vi "Initialization_ITC503_ver1.0.vi"(2 "error in":errorcluster, 3 "Temperature Control (ITC 503):":T1={"GPIB ADR"=0, "Change Heater?"={"Change Heater?"=FALSE, "Heater"=0}, "Change Temp?"={"Change Temp?"=FALSE, "Set Temp (K)"=0.0}, "Cluster"={"Heat Auto?"=FALSE, "Manual Heat?"=FALSE, "Heater Manual (%)"=0.0}, "Change PID?"={"Change PID?"=FALSE, "Proportional"=0.0, "Integral"=0.0, "Derivative"=0.0}, "Change Para?"=FALSE, "ITC503 Control Sensor"=1} {"ITC503 Control Sensor" items=["T2", "T3"]; "Change PID?"."Derivative" format="%.2f"; "Change PID?"."Integral" format="%.2f"; "Change PID?"."Proportional" format="%.2f"; "Cluster"."Heater Manual (%)" scale=0.0..100.0; "Change Temp?"."Set Temp (K)" format="%.3f"; "Change Heater?"."Heater" items=["Heater 1", "Heater 2", "Heater 3"]; "GPIB ADR" items=["None"=0, "24"=24]}) -> (0 "error out":errorcluster, 1 "Temperature Control (ITC 503): 2":T1={"GPIB ADR"=0, "Change Heater?"={"Change Heater?"=FALSE, "Heater"=0}, "Change Temp?"={"Change Temp?"=FALSE, "Set Temp (K)"=0.0}, "Cluster"={"Heat Auto?"=FALSE, "Manual Heat?"=FALSE, "Heater Manual (%)"=0.0}, "Change PID?"={"Change PID?"=FALSE, "Proportional"=0.0, "Integral"=0.0, "Derivative"=0.0}, "Change Para?"=FALSE, "ITC503 Control Sensor"=1} {"ITC503 Control Sensor" items=["T2", "T3"]; "Change PID?"."Derivative" format="%.2f"; "Change PID?"."Integral" format="%.2f"; "Change PID?"."Proportional" format="%.2f"; "Cluster"."Heater Manual (%)" scale=0.0..100.0; "Change Temp?"."Set Temp (K)" format="%.3f"; "Change Heater?"."Heater" items=["Heater 1", "Heater 2", "Heater 3"]; "GPIB ADR" items=["None"=0, "24"=24]})   [LabVIEW 2012]
uses:
  Oxford_itc503/BUSGEN.LLB/OxfordAddress.ctl
panel:
  in  "Delay Time (s)":dbl=1.0
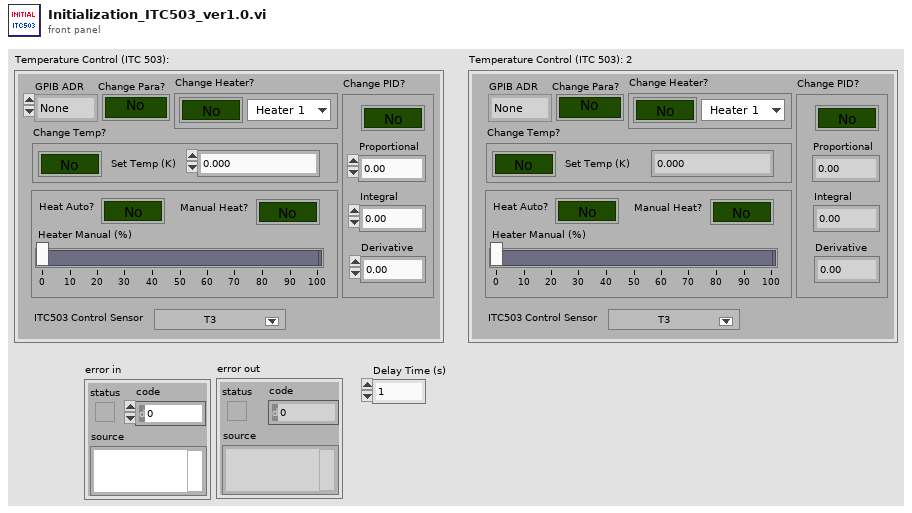
[diagram p1: front panel]
types:
  T1 = cluster{"GPIB ADR":u16, "Change Heater?":cluster{"Change Heater?":bool, "Heater":u8}, "Change Temp?":cluster{"Change Temp?":bool, "Set Temp (K)":dbl}, "Cluster":cluster{"Heat Auto?":bool, "Manual Heat?":bool, "Heater Manual (%)":dbl}, "Change PID?":cluster{"Change PID?":bool, "Proportional":dbl, "Integral":dbl, "Derivative":dbl}, "Change Para?":bool, "ITC503 Control Sensor":u16}
  T2 = typedef "OxfordAddress.ctl" = cluster{"Com Port":i32, "ISOBUS Address":i32, "GPIB Address":i16, "Communication":enum16{"RS232", "ISOBUS", "GPIB", "Gateway"}}
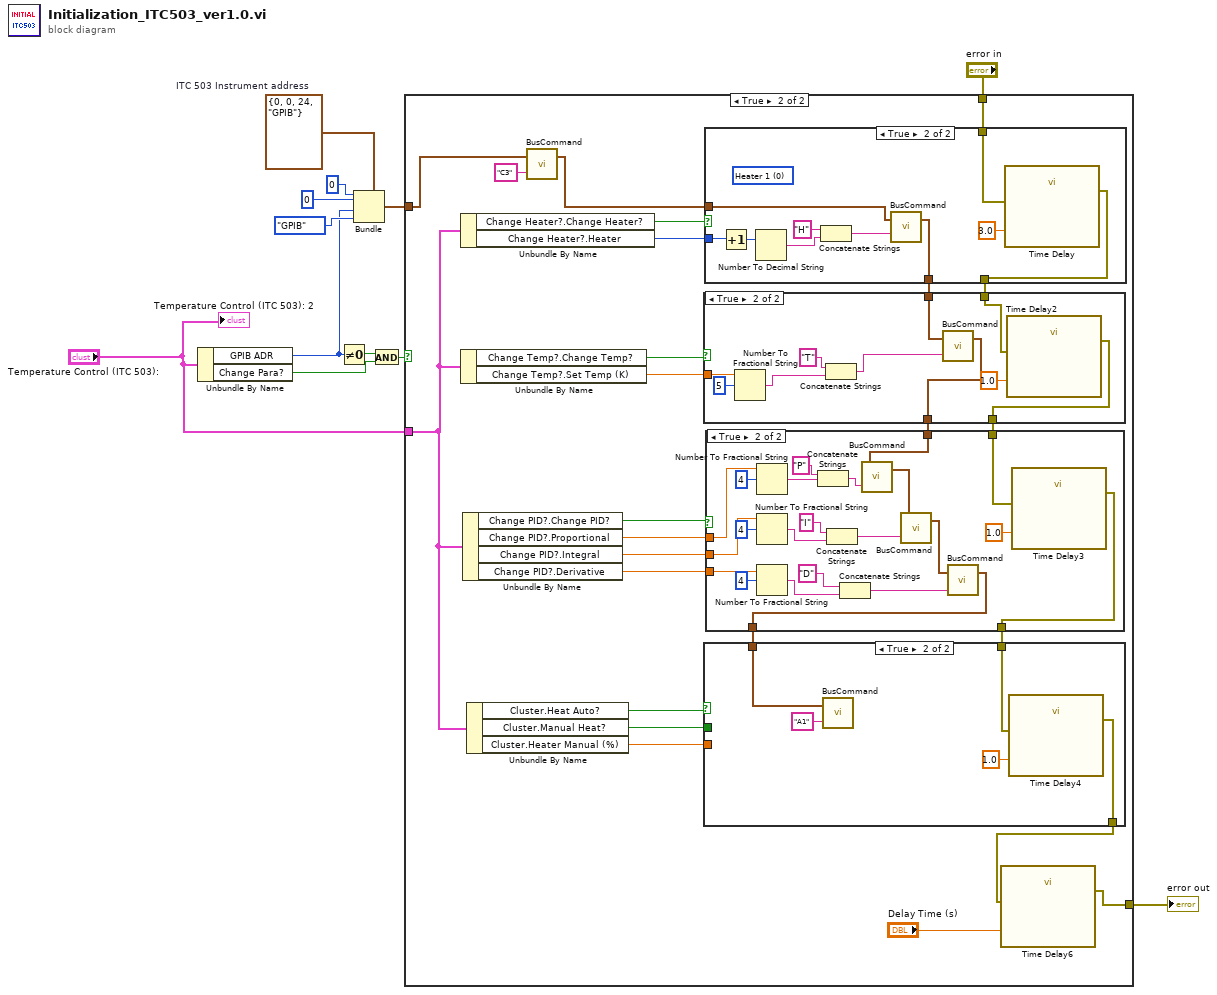
[diagram p0: block diagram]
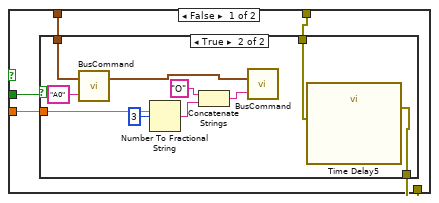
[diagram p3: hidden frame]
diagram:
  w12 = T2 {"Com Port"=0, "ISOBUS Address"=0, "GPIB Address"=24, "Communication"=enum."GPIB"}  # ITC 503 Instrument address
  n1 = Unbundle By Name("Temperature Control (ITC 503):") -> ("GPIB ADR"=w8:u16, "Change Para?"=w6:bool)
  n2 = Not Equal To 0?(x=w8) -> (x != 0?=w5:bool)
  n3 = Bundle(cluster=w12, "Com Port"=0, "ISOBUS Address"=0, "GPIB Address"=w8, "Communication"=enum16{"RS232", "ISOBUS", "GPIB", "Gateway"}."GPIB") -> (w7:T2)
  n4 = And(x=w5, y=w6) -> (x .and. y?=w4:bool)
  n5 = case shown="True" w4 {
    tunnel: w7 -> [_ w24]
    tunnel: "Temperature Control (ITC 503):" -> [_ w29]
    tunnel: "error in" -> [w13 w21]
    tunnel: [w13 w16] -> w2
    frame False {
    }
    frame True {
      n6 = Unbundle By Name(w29) -> ("Change Heater?.Change Heater?"=w38:bool, "Change Heater?.Heater"=w37:u8)
      n7 = Unbundle By Name(w29) -> ("Change Temp?.Change Temp?"=w36:bool, "Change Temp?.Set Temp (K)"=w14:dbl)
      n8 = Unbundle By Name(w29) -> ("Change PID?.Change PID?"=w34:bool, "Change PID?.Proportional"=w33:dbl, "Change PID?.Integral"=w32:dbl, "Change PID?.Derivative"=w31:dbl)
      n9 = Unbundle By Name(w29) -> ("Cluster.Heat Auto?"=w28:bool, "Cluster.Manual Heat?"=w27:bool, "Cluster.Heater Manual (%)"=w26:dbl)
      n10 = call "BusCommand.vi"("Command"="C3", "Instrument address (in)"=w24) -> ("Instrument address (out)"=w22:T2)  [unwired: 1 out]
      n11 = case shown="True" w38 {
        tunnel: w37 -> [_ w105]
        tunnel: w22 -> [w97 w107]
        tunnel: [w97 w101] -> w35
        tunnel: w21 -> [w96 w100]
        tunnel: [w96 w98] -> w20
        frame False {
        }
        frame True {
          (unwired) u8 0 items=["Heater 1", "Heater 2", "Heater 3"] ("Heater")
          n12 = Increment(x=w105) -> (x+1=w104:u8)
          n13 = Number To Decimal String(number=w104) -> (decimal integer string=w103:string)  [unwired: 1 in]
          n14 = Concatenate Strings("H" ("string"), w103) -> (w102:string)
          n15 = call "BusCommand.vi"("Command"=w102, "Instrument address (in)"=w107) -> ("Instrument address (out)"=w101:T2)  [unwired: 1 out]
          n16 = call "Time Delay"("error in (no error)"=w100, "Delay Time (s)"=3.0) -> ("error out"=w98:errorcluster)  [unwired: 9 in]
        }
      }
      n17 = case shown="True" w36 {
        tunnel: w14 -> [_ w95]
        tunnel: w35 -> [w85 w91]
        tunnel: [w85 w90] -> w30
        tunnel: w20 -> [w84 w88]
        tunnel: [w84 w87] -> w19
        frame False {
        }
        frame True {
          n18 = Number To Fractional String(number=w95, width (-)=i16 5) -> (F-format string=w94:string)  [unwired: 2 in]
          n19 = Concatenate Strings("T" ("string"), w94) -> (w92:string)
          n20 = call "BusCommand.vi"("Command"=w92, "Instrument address (in)"=w91) -> ("Instrument address (out)"=w90:T2)  [unwired: 1 out]
          n21 = call "Time Delay2"("error in (no error)"=w88, "Delay Time (s)"=1.0) -> ("error out"=w87:errorcluster)  [unwired: 9 in]
        }
      }
      n22 = case shown="True" w34 {
        tunnel: w33 -> [_ w83]
        tunnel: w32 -> [_ w82]
        tunnel: w31 -> [_ w81]
        tunnel: w30 -> [w61 w80]
        tunnel: [w61 w68] -> w25
        tunnel: w19 -> [w60 w64]
        tunnel: [w60 w63] -> w18
        frame False {
        }
        frame True {
          n23 = Number To Fractional String(number=w83, width (-)=i16 4) -> (F-format string=w78:string)  [unwired: 2 in]
          n24 = Number To Fractional String(number=w82, width (-)=i16 4) -> (F-format string=w74:string)  [unwired: 2 in]
          n25 = Number To Fractional String(number=w81, width (-)=i16 4) -> (F-format string=w72:string)  [unwired: 2 in]
          n26 = Concatenate Strings("P" ("string"), w78) -> (w77:string)
          n27 = Concatenate Strings("I" ("string"), w74) -> (w70:string)
          n28 = Concatenate Strings("D" ("string"), w72) -> (w69:string)
          n29 = call "BusCommand.vi"("Command"=w77, "Instrument address (in)"=w80) -> ("Instrument address (out)"=w76:T2)  [unwired: 1 out]
          n30 = call "BusCommand.vi"("Command"=w70, "Instrument address (in)"=w76) -> ("Instrument address (out)"=w71:T2)  [unwired: 1 out]
          n31 = call "BusCommand.vi"("Command"=w69, "Instrument address (in)"=w71) -> ("Instrument address (out)"=w68:T2)  [unwired: 1 out]
          n32 = call "Time Delay3"("error in (no error)"=w64, "Delay Time (s)"=1.0) -> ("error out"=w63:errorcluster)  [unwired: 9 in]
        }
      }
      n33 = case shown="True" w28 {
        tunnel: w27 -> [w43 _]
        tunnel: w26 -> [w42 _]
        tunnel: w25 -> [w41 w59]
        tunnel: w18 -> [w40 w57]
        tunnel: [w39 w56] -> w17
        frame False {
          n34 = case shown="True" w43 {
            tunnel: w42 -> [_ w54]
            tunnel: w41 -> [_ w49]
            tunnel: w40 -> [w44 w46]
            tunnel: [w44 w45] -> w39
            frame False {
            }
            frame True {
              n35 = call "BusCommand.vi"("Command"="A0", "Instrument address (in)"=w49) -> ("Instrument address (out)"=w50:T2)  [unwired: 1 out]
              n36 = Number To Fractional String(number=w54, width (-)=i16 3) -> (F-format string=w53:string)  [unwired: 2 in]
              n37 = Concatenate Strings("O" ("string"), w53) -> (w51:string)
              n38 = call "BusCommand.vi"("Command"=w51, "Instrument address (in)"=w50) -> ()  [unwired: 2 out]
              n39 = call "Time Delay5"("error in (no error)"=w46) -> ("error out"=w45:errorcluster)  [unwired: 10 in]
            }
          }
        }
        frame True {
          n40 = call "BusCommand.vi"("Command"="A1", "Instrument address (in)"=w59) -> ()  [unwired: 2 out]
          n41 = call "Time Delay4"("error in (no error)"=w57, "Delay Time (s)"=1.0) -> ("error out"=w56:errorcluster)  [unwired: 9 in]
        }
      }
      n42 = call "Time Delay6"("error in (no error)"=w17, "Delay Time (s)"="Delay Time (s)") -> ("error out"=w16:errorcluster)  [unwired: 9 in]
    }
  }
  "error out" <- w2
  "Temperature Control (ITC 503): 2" <- "Temperature Control (ITC 503):"
